vi "remove.volume.vi"(10 "Path":path, 11 "manager_daemon in":refnum<class "manager_daemon.lvclass">) -> (3 "manager_daemon out":refnum<class "manager_daemon.lvclass">)   [LabVIEW 2024, in "manager_daemon.lvclass"]
uses:
  manager_daemon.lvclass
  manager_daemon.lvclass/manager_daemon.ctl
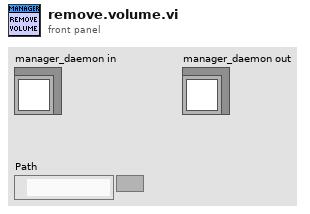
[diagram p1: front panel]
types:
  T1 = map{string, set{cluster{"id":i32, "role":string}}}
  T2 = typedef "manager_daemon.lvclass/sub-map--map.ctl" = map{string, T3}
  T3 = typedef "manager_daemon.lvclass/SubData--cluster.ctl" = cluster{"id":i32, "issues":set{i32}}
  T4 = typedef "manager_daemon.lvclass/IssueData--clustrer.ctl" = cluster{"cover_date":timestamp, "cv_id":string, "name":string, "sortable_name":string, "issue_number":string, "deck":string, "description":string, "id":i32, "store_date":timestamp, "date_last_updated":timestamp, "site_detail_url":string, "cover_url":string, "source_path":path, "character map":map{i32, string}, "concept map":map{i32, string}, "storyArc map":map{i32, string}, "team map":map{i32, string}, "creator map":map{i32, cluster{"name":string, "role":string}}}
  T5 = typedef "manager_daemon.lvclass/VolumeData--cluster.ctl" = cluster{"name":string, "sortable_name":string, "aliases":string[], "description":string, "site_detail_url":string, "count_of_issues":i32, "start_year":i32, "publisher_id":i32, "issue_ids":i32[], "date_last_updated":timestamp, "volume":i32, "cv_id":string, "volume type":T6, "source_path":path}
  T6 = typedef "CV_Shared_Library.lvlib/volume.type--enum.ctl" = enum16{"Ongoing", "Limited Series", "Annual", "One Shot", "Reprint/Document", "Star Comics", "Epic Comics"}
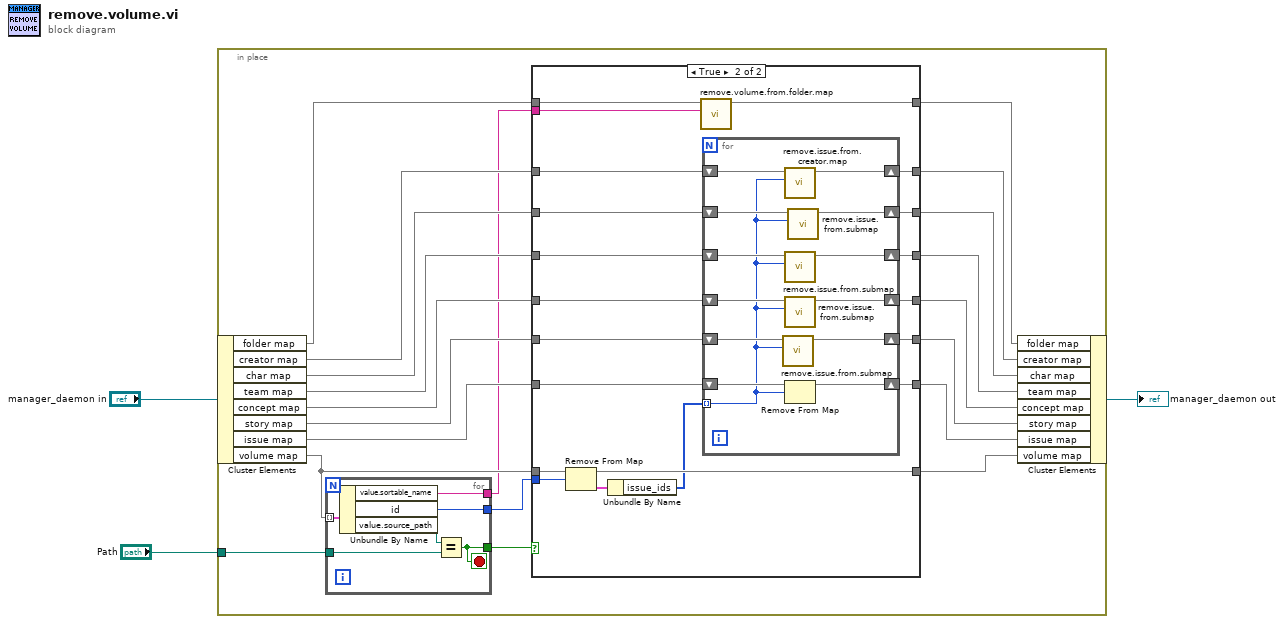
[diagram p0: block diagram]
diagram:
  n1 = in-place {
    in-place-border: "Path" -> [w23]
    n2 = in-place-cluster #1("manager_daemon in") -> ("folder map"=w5:map{i32, map{string, i32}}, "creator map"=w8:T1, "char map"=w13:T2, "team map"=w14:T2, "concept map"=w15:T2, "story map"=w16:T2, "issue map"=w18:map{i32, T4}, "volume map"=w22:map{i32, T5})
    n3 = for {
      tunnel: w22 -> [w70] mode=indexing
      tunnel: w23 -> [w68]
      tunnel: [w67] -> w20
      tunnel: [w66] -> w19
      tunnel: [w65] -> w6
      stop <- w66 stop-if-true
      n4 = Unbundle By Name(w70) -> ("value.sortable_name"=w65:string, "id"=w67:i32, "value.source_path"=w69:path)
      n5 = Equal?(x=w69, y=w68) -> (x = y?=w66:bool)
    }
    n6 = case shown="True" w19 {
      tunnel: w22 -> [w31 w51]
      tunnel: [w31 w50] -> w21
      tunnel: w20 -> [_ w49]
      tunnel: w18 -> [w30 w47]
      tunnel: [w30 w46] -> w17
      tunnel: w16 -> [w29 w44]
      tunnel: w15 -> [w28 w43]
      tunnel: w14 -> [w27 w42]
      tunnel: w13 -> [w26 w41]
      tunnel: [w29 w40] -> w12
      tunnel: [w28 w39] -> w11
      tunnel: [w27 w38] -> w10
      tunnel: [w26 w37] -> w9
      tunnel: w8 -> [w25 w36]
      tunnel: [w25 w35] -> w7
      tunnel: w6 -> [_ w32]
      tunnel: w5 -> [w24 w34]
      tunnel: [w24 w33] -> w4
      frame False {
      }
      frame True {
        n7 = Remove From Map(10:w49, 11:w51) -> (1:w48:T5, 3:w50:map{i32, T5})  [unwired: 1 out]
        n8 = Unbundle By Name(w48) -> ("issue_ids"=w45:i32[])
        n9 = call "remove.volume.from.folder.map.vi"("sortable name"=w32, "folder map in"=w34) -> ("folder map out"=w33:map{i32, map{string, i32}})  [unwired: 9 in]
        n10 = for {
          shift-right: [w63] -> w46
          shift-left: w47 -> [w64]
          tunnel: w45 -> [w53] mode=indexing
          shift-right: [w61] -> w40
          shift-left: w44 -> [w62]
          shift-right: [w57] -> w39
          shift-left: w43 -> [w60]
          shift-right: [w56] -> w38
          shift-left: w42 -> [w59]
          shift-right: [w55] -> w37
          shift-left: w41 -> [w58]
          shift-right: [w52] -> w35
          shift-left: w36 -> [w54]
          n11 = call "remove.issue.from.submap.vi"("issue id"=w53, "map in"=w62) -> ("map out"=w61:T2)  [unwired: 9 in]
          n12 = call "remove.issue.from.creator.map.vi"("issue id"=w53, "creator map in"=w54) -> ("creator map out"=w52:T1)  [unwired: 9 in]
          n13 = call "remove.issue.from.submap.vi"("issue id"=w53, "map in"=w59) -> ("map out"=w56:T2)  [unwired: 9 in]
          n14 = call "remove.issue.from.submap.vi"("issue id"=w53, "map in"=w60) -> ("map out"=w57:T2)  [unwired: 9 in]
          n15 = Remove From Map(10:w53, 11:w64) -> (3:w63:map{i32, T4})  [unwired: 2 out]
          n16 = call "remove.issue.from.submap.vi"("issue id"=w53, "map in"=w58) -> ("map out"=w55:T2)  [unwired: 9 in]
        }
      }
    }
    n17 = in-place-cluster #1("folder map"=w4, "creator map"=w7, "char map"=w9, "team map"=w10, "concept map"=w11, "story map"=w12, "issue map"=w17, "volume map"=w21) -> (→"manager_daemon out":refnum<class "manager_daemon.lvclass">)
  }
